vi "Get gRPC Device Server Location.vi"(8 "error in":errorcluster, 10 "session name":string, 11 "instrument in":refnum<class "ISession Factory.lvclass">) -> (0 "error out":errorcluster, 1 "using device service":bool, 2 "remote connection options":T1, 3 "instrument out":refnum<class "ISession Factory.lvclass">, 4 "location unique id":u64)   [LabVIEW 2021, in "NI Session Management V1 Client.lvlib" / "Session Reservation.lvclass"]
uses:
  Session Reservation.lvclass
  Sessions/Instrument/ISession Factory/ISession Factory.lvclass
  Sessions/Instrument/ISession Factory/Remote Connection Options.ctl
  Discovery V1/TypeDefs/Service Location FGV Action.ctl
  gRPC/Generated APIs/ni/measurementlink/discovery/v1/RPC Messages/ni_measurementlink_discovery_v1_ResolveServiceRequest.ctl
  Session Reservation.lvclass/Session Reservation.ctl
  Discovery V1/NI Discovery V1 Client.lvlib
  gRPC/Generated APIs/ni/measurementlink/discovery/v1/ni.measurementlink.discovery.v1.api.lvlib
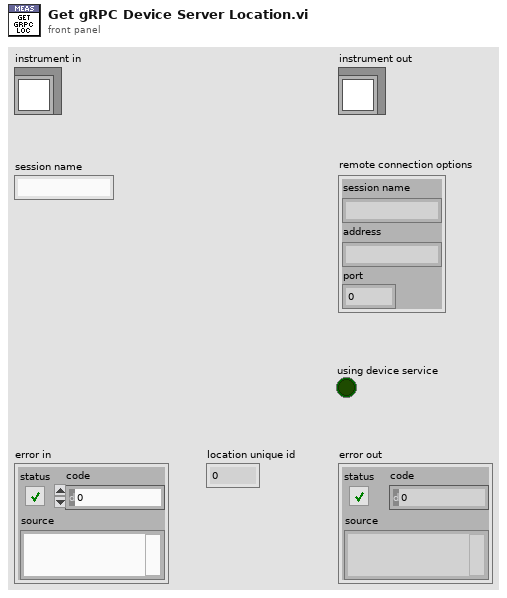
[diagram p1: front panel]
types:
  T1 = typedef "NI Session Management Instrument.lvlib/ISession Factory.lvclass/Remote Connection Options.ctl" = cluster{"session name":string, "address":string, "port":u32}
  T2 = typedef "ni.measurementlink.discovery.v1.api.lvlib/ni_measurementlink_discovery_v1_ResolveServiceRequest.ctl" = cluster{"provided_interface":string, "service_class":string, "deployment_target":string, "version":string}
  T3 = typedef "NI Discovery V1 Client.lvlib/Service Location FGV Action.ctl" = enum16{"Get Service Location", "Reresolve Service Location"}
  T4 = typedef "ni.measurementlink.discovery.v1.api.lvlib/ni_measurementlink_discovery_v1_ServiceLocation.ctl" = cluster{"location":string, "insecure_port":string, "ssl_authenticated_port":string}
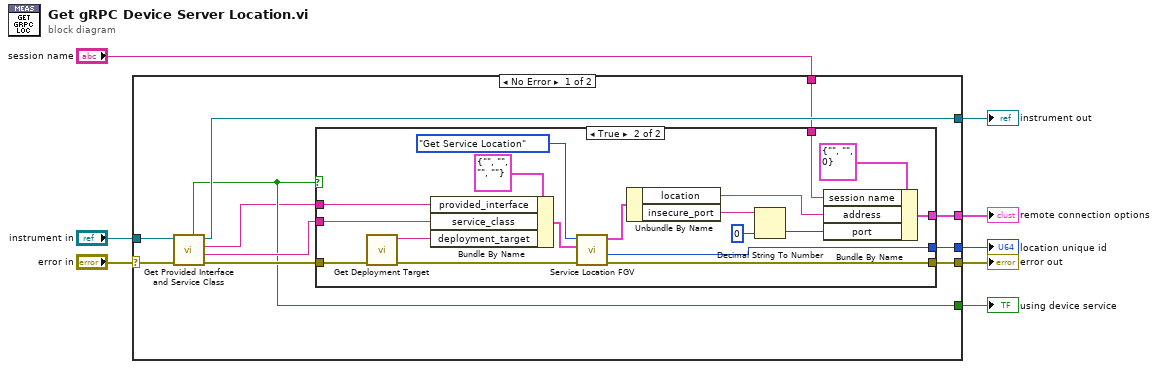
[diagram p0: block diagram]
diagram:
  n1 = case shown="No Error" "error in" {
    selector: "error in" -> [w15 w40]
    tunnel: [w19 w40] -> w8
    tunnel: [w18 w39] -> w7
    tunnel: "instrument in" -> [w16 w39]
    tunnel: [w14 _] -> w4
    tunnel: "session name" -> [w13 _]
    tunnel: [w11 _] -> w2
    tunnel: [w10 _] -> w1
    frame No Error {
      n2 = call "Get Provided Interface and Service Class.vi"("error in"=w15, "instrument in"=w16) -> ("error out"=w17:errorcluster, "service class"=w12:string, "provided interface"=w9:string, "instrument out"=w18:refnum<class "ISession Factory.lvclass">, "using device service"=w11:bool)  [unwired: 5 in]
      n3 = case shown="True" w11 {
        tunnel: [w20 w35] -> w19
        tunnel: w12 -> [_ w34]
        tunnel: w9 -> [_ w33]
        tunnel: w17 -> [w20 w22]
        tunnel: [_ w26] -> w14
        tunnel: w13 -> [_ w25]
        tunnel: [_ w24] -> w10
        frame False {
        }
        frame True {
          n4 = call "Get Deployment Target.vi"("error in (no error)"=w22) -> ("error out"=w23:errorcluster, "deployment_target"=w21:string)  [unwired: 9 in]
          n5 = Bundle By Name(cluster=T2 {"provided_interface"="", "service_class"="", "deployment_target"="", "version"=""} ("Resolve Service Request"), "provided_interface"=w33, "service_class"=w34, "deployment_target"=w21) -> (w30:T2)
          n6 = call "Service Location FGV.vi"("error in"=w23, "resolve service request"=w30, "action"=Service_Location_FGV_Action."Get Service Location" ("Action")) -> ("error out"=w35:errorcluster, "location unique id out"=w24:u64, "service location"=w37:T4)  [unwired: 6 in]
          n7 = Unbundle By Name(w37) -> ("location"=w28:string, "insecure_port"=w36:string)
          n8 = Decimal String To Number(string=w36, default (0L)=u32 0 ("default (0 I32)")) -> (number=w27:u32)  [unwired: 1 in, 1 out]
          n9 = Bundle By Name(cluster=T1 {"session name"="", "address"="", "port"=0} ("remote connection options"), "session name"=w25, "address"=w28, "port"=w27) -> (w26:T1)
        }
      }
    }
    frame Error {
    }
  }
  "error out" <- w8
  "instrument out" <- w7
  "remote connection options" <- w4
  "using device service" <- w2
  "location unique id" <- w1
